vi "access insert core.vi"(5 "data":variant[](array[variant]), 6 "delete table?":bool, 7 "columns":string[](array[string]), 8 "error in (no error)":errorcluster, 11 "table":string) -> (0 "error out":errorcluster)   [LabVIEW 2016, in "opSignIn.lvlib"]
uses:
  opSignIn.lvlib
  <vilib>/addons/database/Connection.llb/DB Tools Open Connec (String).vi
  <vilib>/addons/database/NI_Database_API.lvlib
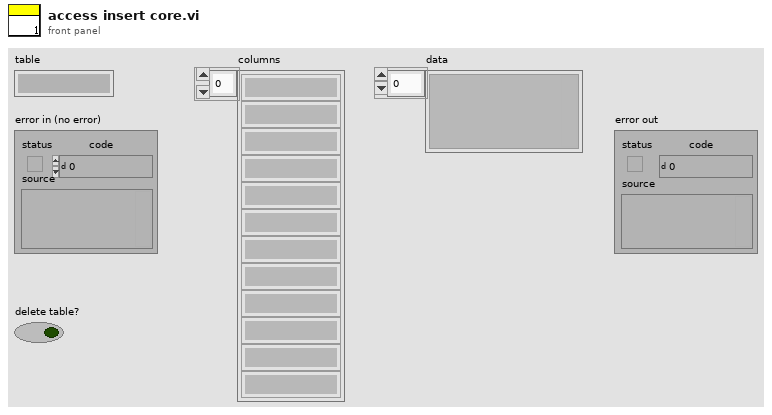
[diagram p1: front panel]
types:
  T1 = typedef "NI_Database_API.lvlib/Conn ObjectReference.ctl" = refnum<k1>
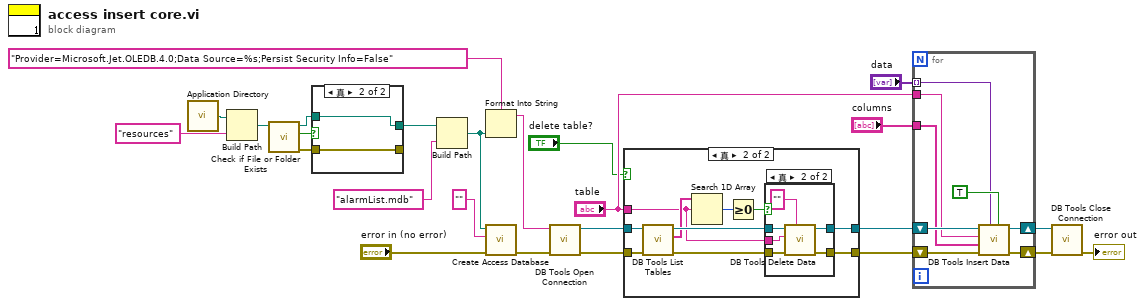
[diagram p0: block diagram]
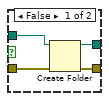
[diagram p4: hidden frame]
diagram:
  n1 = call <vilib>:"Application Directory.vi"() -> ("Application Directory"=w19:path)
  n2 = Build Path(base path=w19, name or relative path="resources" ("名称或相对路径")) -> (appended path=w17:path)
  n3 = call <vilib>:"Check if File or Folder Exists.vi"("path"=w17) -> ("error out"=w14:errorcluster, "file or folder exists?"=w16:bool, "dup path"=w15:path)  [unwired: 8 in]
  n4 = case shown="真" w16 {
    tunnel: [w26 w31] -> w13
    tunnel: w15 -> [w29 w31]
    tunnel: w14 -> [w28 w30]
    tunnel: [w27 w30] -> _
    frame False {
      n5 = Create Folder(path (use dialog)=w29, error in=w28) -> (created path=w26:path, error out=w27:errorcluster)  [unwired: 1 in, 1 out]
    }
    frame True {
    }
  }
  n6 = Build Path(base path=w13, name or relative path="alarmList.mdb" ("名称或相对路径")) -> (appended path=w11:path)
  n7 = Format Into String(format string="Provider=Microsoft.Jet.OLEDB.4.0;Data Source=%s;Persist Security Info=False", w11) -> (resulting string=w22:string)  [unwired: 2 in, 1 out]
  n8 = call "Create Access Database.vi"("错误输入（无错误）"="error in (no error)", "Password"="", "路径"=w11) -> ("错误输出"=w21:errorcluster)  [unwired: 8 in]
  n9 = call-poly <vilib>:"DB Tools Open Connection.vi"("error in (no error)"=w21, "connection information"=w22) -> ("error out"=w4:errorcluster, "connection reference"=w6:T1)  [unwired: 6 in]
  n10 = case shown="真" "delete table?" {
    tunnel: w6 -> [w33 w39]
    tunnel: [w33 w43] -> w5
    tunnel: w4 -> [w32 w42]
    tunnel: [w32 w41] -> w3
    tunnel: "table" -> [_ w36]
    frame False {
    }
    frame True {
      n11 = call <vilib>:"DB Tools List Tables.vi"("error in (no error)"=w42, "connection reference"=w39) -> ("error out"=w40:errorcluster, "tables"=w37:string[], "connection reference out"=w38:T1)  [unwired: 3 in]
      n12 = Search 1D Array(1D array=w37, element=w36) -> (index of element=w35:i32)  [unwired: 1 in]
      n13 = Greater Or Equal To 0?(x=w35) -> (x >= 0?=w34:bool)
      n14 = case shown="真" w34 {
        tunnel: [w45 w51] -> w43
        tunnel: [w44 w50] -> w41
        tunnel: w40 -> [w44 w49]
        tunnel: w38 -> [w45 w48]
        tunnel: w36 -> [_ w47]
        frame False {
        }
        frame True {
          n15 = call <vilib>:"DB Tools Delete Data.vi"("condition"="", "error in (no error)"=w49, "table"=w47, "connection reference"=w48) -> ("error out"=w50:errorcluster, "connection reference out"=w51:T1)  [unwired: 6 in]
        }
      }
    }
  }
  n16 = for {
    shift-right: [w56] -> w24
    shift-left: w3 -> [w59]
    shift-right: [w57] -> w25
    shift-left: w5 -> [w58]
    tunnel: "columns" -> [w54]
    tunnel: "table" -> [w53]
    tunnel: "data" -> [w52] mode=indexing
    n17 = call <vilib>:"DB Tools Insert Data.vi"("create table? (F)"=TRUE, "data"=w52, "error in (no error)"=w59, "columns"=w54, "table"=w53, "connection reference"=w58) -> ("error out"=w56:errorcluster, "connection reference out"=w57:T1)  [unwired: 4 in]
  }
  n18 = call <vilib>:"DB Tools Close Connection.vi"("error in (no error)"=w24, "connection reference"=w25) -> ("error out"=→"error out":errorcluster)  [unwired: 5 in]
